vi "Write Timeout.vi"(8 "Error In":errorcluster, 10 "Timeout":i32, 11 "Session In":refnum<class "Session.lvclass">) -> (0 "Error Out":errorcluster, 3 "Sesssion Out":refnum<class "Session.lvclass">)   [LabVIEW 2021, in "Field_RnD_Services_LIBSSH2_Toolkit.lvlib" / "Session.lvclass"]
doc: "Sets the timeout in milliseconds (ms) for reading and writing during the communication with a remote SSH/SFTP server."
uses:
  Session.lvclass
  Session.lvclass/Session.ctl
  Field_RnD_Services_LIBSSH2_Toolkit.lvlib
  SSH/SSH.lvclass
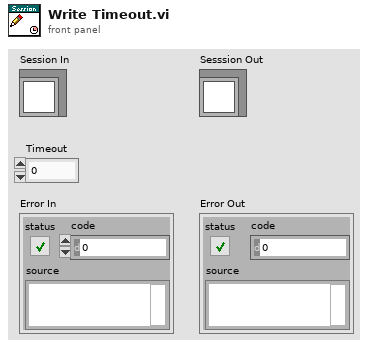
[diagram p1: front panel]
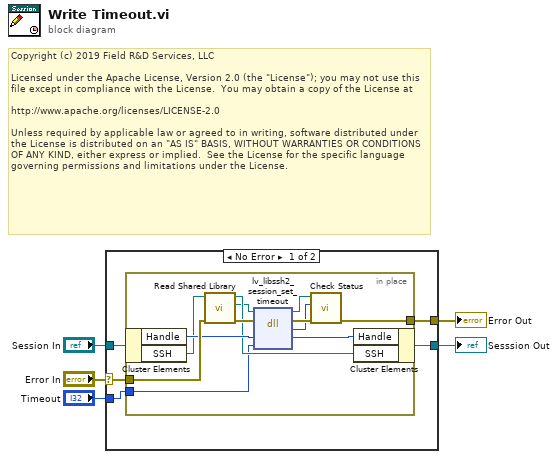
[diagram p0: block diagram]
diagram:
  # "Copyright (c) 2019 Field R&D Services, LLC\n\nLicensed under the Apache License, Version 2.0 (the \"License\"); you may not use this file except in compliance with the License.  You may obtain a copy of the License at\n\nhttp://www.apache.org/licenses/LICENSE-2.0\n\nUnless required by applicable law or agreed to in writing, software distributed under the License is distributed on an \"AS IS\" BASIS, WITHOUT WARRANTIES OR CONDITIONS OF ANY KIND, either express or implied.  See the License for the specific language governing permissions and limitations under the License."
  n1 = case shown="No Error" "Error In" {
    selector: "Error In" -> [w9 w24]
    tunnel: [w10 w24] -> w4
    tunnel: "Session In" -> [w8 w23]
    tunnel: [w7 w23] -> w2
    tunnel: "Timeout" -> [w6 _]
    frame No Error {
      n2 = in-place {
        in-place-border: [w18] -> w10
        in-place-border: w9 -> [w22]
        in-place-border: w6 -> [w11]
        n3 = in-place-cluster #1(w8) -> ("Handle"=w21:u64, "SSH"=w14:refnum<class "SSH.lvclass">)
        n4 = call "Read Shared Library.vi"("Error In"=w22, "SSH In"=w14) -> ("Error Out"=w15:errorcluster, "libssh2lv Shared Library"=w12:path, "SSH Out"=w13:refnum<class "SSH.lvclass">)  [unwired: 7 in]
        n5 = dll-call lib="D:/Users/cfield/Code/Field R&D Services/SSH/libssh2-labview/src/Toolkit/Support/libssh2lv.*" fn="lv_libssh2_session_set_timeout"(path in=w12, error in=w15, "session"=w21, "milliseconds"=w11) -> (path out=w17:path, error out=w19:errorcluster, "status"=w16:i32, "session"=w20:u64)  [unwired: 2 in]
        n6 = call "Check Status.vi"("Error In"=w19, "Status"=w16, "libssh2lv Shared Library In"=w17) -> ("Error Out"=w18:errorcluster)  [unwired: 7 in, 1 out]
        n7 = in-place-cluster #1("Handle"=w20, "SSH"=w13) -> (w7:refnum<class "Session.lvclass">)
      }
    }
    frame Error {
    }
  }
  "Sesssion Out" <- w2
  "Error Out" <- w4
